vi "RobotMap.vi"() -> ()   [LabVIEW 2018]
panel:
  in  "4Bar Limit Switch BottomDIO":dbl
  in  "RightDriveSlave2":u8=10
  in  "LeftDriveSlave2":u8=3
  in  "Cargo Intake":dbl=5.0
  in  "Hatch Panel Intake":dbl=6.0
  in  "4BarSlave":u8=7
  in  "4BarMaster":u8=4
  in  "RightDriveSlave1":u8=9
  in  "RightDriveMaster":u8=8
  in  "LeftDriveSlave1":u8=2
  in  "LeftDriveMaster":u8=1
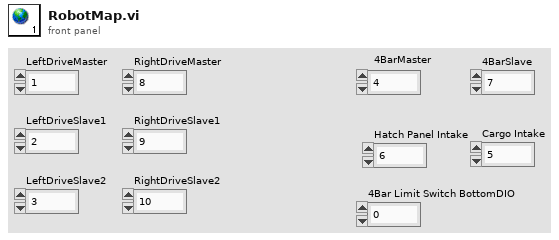
[diagram p1: front panel]
diagram:
